vi "Measurement Logic.vi"() -> ()   [LabVIEW 2022 SP3, in "Calibrate Acoustic Output Level.lvlib"]
uses:
  Calibrate Acoustic Output Level.lvlib
  <vilib>/Plug-In SDKs/Measurements/Measure Call Context/Measure Call Context.lvclass
  Measurement Configuration.ctl
  Measurement Results.ctl
  <vilib>/addons/_NISVFA/_Generation/Signal Generation/SV Signal/sv_System Timing Model.ctl
  <vilib>/DAQmx/write.llb/DAQmx Write (Analog Wfm 1Chan NSamp).vi
  <vilib>/Analysis/1siggen.llb/Ramp Pattern by Samples.vi
  <vilib>/addons/_NISVFA/_Generation/Signal Generation/SV Sinusoid/SV Sinusoid.lvclass
  C:/Program Files/National Instruments/LabVIEW 2022/vi.lib/addons/_NISVFA/_Generation/Signal Generation/SV Signal/SV Signal.lvclass
  <vilib>/addons/_NISVFA/_Generation/Signal Generation/SV Sinusoid/Configure Sine.vi
  <vilib>/DAQmx/create/channels.llb/DAQmx Create Channel (AO-Voltage-Basic).vi
  <vilib>/DAQmx/configure/timing.llb/DAQmx Timing (Sample Clock).vi
  <vilib>/addons/_NISVFA/_Generation/Signal Generation/SV Signal/Write Sample Rate.vi
  <vilib>/addons/_NISVFA/_Generation/Signal Generation/SV Signal/Write System Timing Model.vi
  <vilib>/addons/_NISVFA/_Generation/Signal Generation/SV Signal/Write Ramp Parameters.vi
  <vilib>/DAQmx/miscellaneous.llb/DAQmx Fill In Error Info.vi
  <vilib>/DAQmx/create/channels.llb/DAQmx Create Channel (AI-Sound Pressure-Microphone).vi
  <vilib>/addons/_NISVFA/_Generation/Signal Generation/SV Signal/SV Signal.lvclass
  <vilib>/addons/Sound and Vibration/svt_Level/SoundVib_SoundLevel.lvlib
  <resource>/objmgr/daqmx.rc
  <vilib>/Analysis/NI_AALBase.lvlib
  <vilib>/gmath/NI_Gmath.lvlib
  <vilib>/addons/Sound and Vibration/svt_Level/SVL Leq Sound Level (1 Ch).vi
  <vilib>/DAQmx/read.llb/DAQmx Read (Analog Wfm 1Chan NSamp).vi
panel:
  out "crossed":bool=TRUE
  out "output voltage ratio":dbl=3.3942875477425276 format="%#_g Pa/Vpk"
  out "Waveform Graph":waveform(dbl)(graph)={"t0"=timestamp(3812465362.0113354 s since 1904-01-01), "dt"=1.9531249997269942e-05, "Y"=array[12800 elements], "attributes"=variant("NI_ChannelName"=variant(string "PXI1Slot2/ai0"), "NI_UnitDescription"=variant(string "Pascals"), "NI_dBReference"=variant(dbl 2e-05))}
  out "dBSPL":dbl=98.44719956931596
  out "measurement results":T1
  in  "measurement configuration":T2={"output channel"="Lorem ipsum dolor sit", "target value (dB)"=1.2, "number of steps"=32.0, "start amplitude (Vpk)"=32.0, "stop amplitude (Vpk)"=64.0, "frequency"=64.0, "ref mic channel"="PXI1Slot3\\ai0", "ref mic sensitivity (mV/Pa)"=-32.0} {"stop amplitude (Vpk)" format="%#_3f"; "start amplitude (Vpk)" format="%#.3f"}
  out "measure call context out":refnum<class "Measure Call Context.lvclass">
  in  "measure call context in":refnum<class "Measure Call Context.lvclass">
  out "error out":errorcluster
  in  "error in":errorcluster
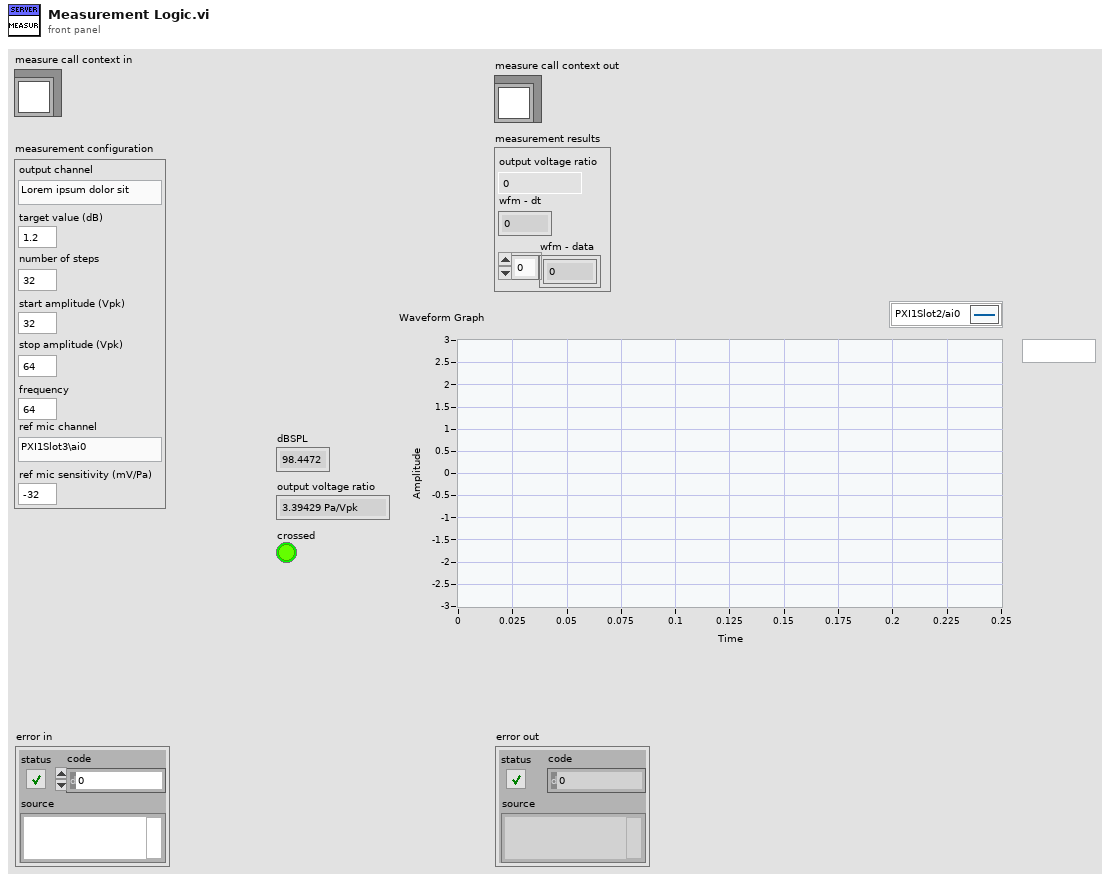
[diagram p1: front panel]
types:
  T1 = typedef "Calibrate Acoustic Output Level.lvlib/Measurement Results.ctl" = cluster{"output voltage ratio":dbl, "wfm - dt":dbl, "wfm - data":dbl[]}
  T2 = typedef "Calibrate Acoustic Output Level.lvlib/Measurement Configuration.ctl" = cluster{"output channel":string, "target value (dB)":dbl, "number of steps":dbl, "start amplitude (Vpk)":dbl, "stop amplitude (Vpk)":dbl, "frequency":dbl, "ref mic channel":string, "ref mic sensitivity (mV/Pa)":dbl}
  T3 = typedef "SV Signal.lvclass/sv_System Timing Model.ctl" = i64
  T4 = cluster{"profile":enum16{"Linear", "Half cosine"}, "durations [s]":cluster{"ramp-up":dbl, "transition":dbl, "ramp-down":dbl}}
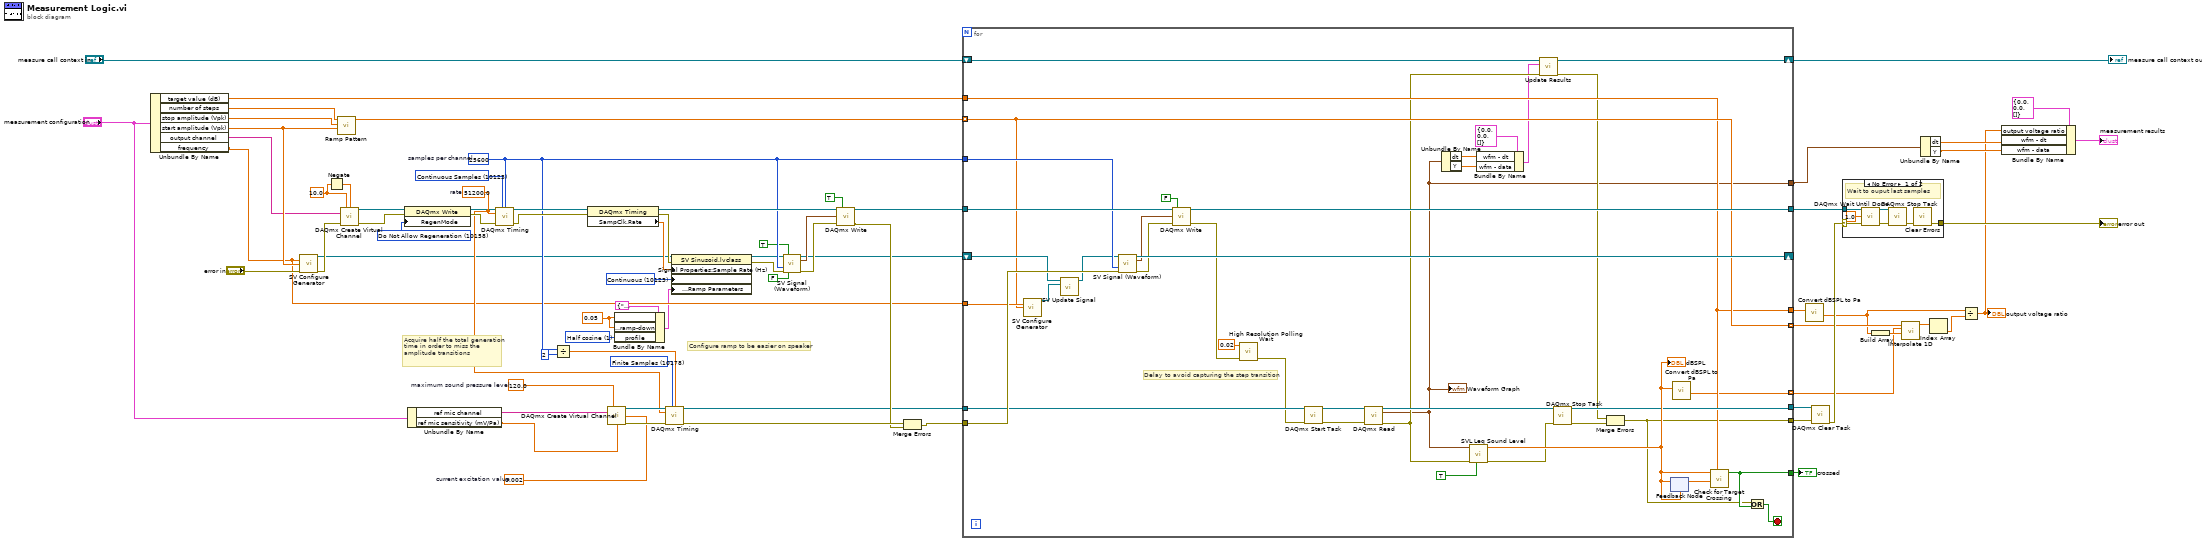
[diagram p0: block diagram]
diagram:
  w8 = 0.05 ("ramp duration")
  w6 = u16 1 items=["Linear", "Half cosine"] ("ramp profile")
  w5 = T3 10123 items=["Finite"=10178, "-"=-1, "Continuous"=10123, "-"=-2, "Settled"=110123, "Averaged"=210123, "Discrete Sweep"=310123, "Continuous Sweep"=410123] ("System Timing Model")
  w51 = 0.002  # current excitation value
  w54 = 120.0  # maximum sound pressure level
  w55 = 10178 items=["Finite Samples"=10178, "Continuous Samples"=10123] ("sample mode")
  w62 = 10158 items=["Allow Regeneration"=10097, "Do Not Allow Regeneration"=10158] ("RegenMode")
  w66 = 10.0 ("maximum value")
  w37 = 25600  # samples per channel
  w68 = 10123 items=["Finite Samples"=10178, "Continuous Samples"=10123, "Hardware Timed Single Point"=12522] ("sample mode")
  w42 = 51200.0  # rate
  # "Configure ramp to be easier on speaker"
  # "Acquire half the total generation time in order to miss the amplitude transitions"
  n1 = Unbundle By Name("measurement configuration") -> ("target value (dB)"=w25:dbl, "number of steps"=w24:dbl, "stop amplitude (Vpk)"=w23:dbl, "start amplitude (Vpk)"=w22:dbl, "output channel"=w21:string, "frequency"=w20:dbl)
  n2 = call-poly <vilib>:"SV Configure Generator.vi"("frequency (Hz)"=w20, "amplitude"=w22, "error in (no error)"="error in") -> ("signal configuration"=w11:refnum<class "SV Sinusoid.lvclass">, "error out"=w64:errorcluster)  [unwired: 11 in]
  n3 = Negate(x=w66) -> (-x=w65:dbl)
  n4 = call-poly <vilib>:"Ramp Pattern.vi"("start"=w22, "end"=w23, "samples"=w24) -> ("Ramp Pattern"=w41:dbl[])  [unwired: 7 in, 1 out]
  n5 = call-poly <vilib>:"DAQmx Create Virtual Channel.vi"("maximum value"=w66, "minimum value"=w65, "physical channels"=w21, "error in"=w64) -> ("task out"=w61:refnum<k21>, "error out"=w59:errorcluster)  [unwired: 10 in]
  n6 = property class="DAQmx Write"(reference=w61, error in=w59, "RegenMode"=w62) -> (reference out=w60:refnum<k21>, error out=w58:errorcluster)
  n7 = Unbundle By Name("measurement configuration") -> ("ref mic channel"=w19:string, "ref mic sensitivity (mV/Pa)"=w18:dbl)
  n8 = call-poly <vilib>:"DAQmx Timing.vi"("task/channels in"=w60, "sample mode"=w68, "samples per channel"=w37, "rate"=w42, "error in"=w58) -> ("task out"=w69:refnum<k21>, "error out"=w67:errorcluster)  [unwired: 9 in]
  n9 = Divide(x=w37, y=2) -> (x/y=w35:dbl)
  n10 = property class="DAQmx Timing"(reference=w69, error in=w67) -> (reference out=w48:refnum<k21>, error out=w56:errorcluster, "SampClk.Rate"=w57:dbl)
  n11 = call-poly <vilib>:"DAQmx Create Virtual Channel.vi"("maximum sound pressure level"=w54, "physical channels"=w19, "current excitation value"=w51, "microphone sensitivity"=w18) -> ("task out"=w53:refnum<k21>, "error out"=w52:errorcluster)  [unwired: 10 in]
  n12 = Bundle By Name(cluster=T4 {"profile"=enum."Linear", "durations [s]"={"ramp-up"=0.0, "transition"=0.0, "ramp-down"=0.0}} ("Ramp Parameters:All Elements"), "durations [s].ramp-up"=w8, "durations [s].ramp-down"=w8, "profile"=w6) -> (w7:T4)
  n13 = call-poly <vilib>:"DAQmx Timing.vi"("task/channels in"=w53, "sample mode"=w55, "samples per channel"=w35, "rate"=w42, "error in"=w52) -> ("task out"=w39:refnum<k21>, "error out"=w45:errorcluster)  [unwired: 9 in]
  n14 = property class="SV Sinusoid.lvclass"(reference=w11, error in=w56, "Signal Properties:Sample Rate (Hz)"=w57, "Signal Properties:System Timing Model"=w5, "Signal Properties:Ramps:Ramp Parameters"=w7) -> (reference out=w4:refnum<class "SV Sinusoid.lvclass">, error out=w3:errorcluster)
  n15 = call-dynamic "SV Signal (Waveform).vi"("signal configuration"=w4, "reset"=TRUE, "samples"=w37, "error in (no error)"=w3, "stop"=FALSE) -> ("signal configuration"=w10:refnum<class "SV Sinusoid.lvclass">, "output waveform"=w49:waveform(dbl), "error out"=w50:errorcluster)  [unwired: 5 in, 3 out]
  n16 = call-poly <vilib>:"DAQmx Write.vi"("task/channels in"=w48, "auto start"=TRUE, "data"=w49, "error in"=w50) -> ("task out"=w47:refnum<k21>, "error out"=w40:errorcluster)  [unwired: 9 in, 1 out]
  n17 = Merge Errors(w45, w40) -> (w38:errorcluster)
  n18 = for {
    shift-right: [w114] -> _
    shift-left: w10 -> [w105]
    tunnel: w37 -> [w108]
    tunnel: w47 -> [w113]
    tunnel: [w112] -> w63
    tunnel: w38 -> [w107]
    tunnel: w39 -> [w98]
    tunnel: [w94] -> w44
    tunnel: w20 -> [w103]
    tunnel: w41 -> [w89] mode=indexing
    tunnel: w25 -> [w88]
    tunnel: [w90] -> w28
    tunnel: [w89] -> w29 mode=indexing
    tunnel: [w87] -> w33 mode=indexing
    tunnel: [w88] -> w32
    shift-right: [w82] -> w71
    shift-left: "measure call context in" -> [w81]
    tunnel: [w76] -> w17
    tunnel: [w75] -> w12
    stop <- w101 stop-if-true
    # "Delay to avoid capturing the step transition"
    n19 = call-poly <vilib>:"SV Configure Generator.vi"("frequency (Hz)"=w103, "amplitude"=w89) -> ("signal configuration"=w106:refnum<class "SV Sinusoid.lvclass">)  [unwired: 12 in, 1 out]
    n20 = call-dynamic "SV Update Signal.vi"("current configuration"=w105, "new configuration"=w106) -> ("updated configuration"=w104:refnum<class "SV Sinusoid.lvclass">)  [unwired: 12 in, 1 out]
    n21 = call-dynamic "SV Signal (Waveform).vi"("signal configuration"=w104, "samples"=w108, "error in (no error)"=w107) -> ("signal configuration"=w114:refnum<class "SV Sinusoid.lvclass">, "output waveform"=w109:waveform(dbl), "error out"=w111:errorcluster)  [unwired: 7 in, 3 out]
    n22 = call-poly <vilib>:"DAQmx Write.vi"("task/channels in"=w113, "auto start"=FALSE, "data"=w109, "error in"=w111) -> ("task out"=w112:refnum<k21>, "error out"=w93:errorcluster)  [unwired: 9 in, 1 out]
    n23 = call <vilib>:"High Resolution Polling Wait.vi"("error in (no error)"=w93, "seconds to wait"=0.02) -> ("error out"=w92:errorcluster)  [unwired: 9 in]
    n24 = call <vilib>:"DAQmx Start Task.vi"("task/channels in"=w98, "error in"=w92) -> ("task out"=w97:refnum<k21>, "error out"=w96:errorcluster)  [unwired: 12 in]
    n25 = call-poly <vilib>:"DAQmx Read.vi"("task/channels in"=w97, "error in"=w96) -> ("task out"=w95:refnum<k21>, "data"=w76:waveform(dbl), "error out"=w85:errorcluster)  [unwired: 11 in]
    "Waveform Graph" <- w76
    n26 = Unbundle By Name(w76) -> ("dt"=w78:dbl, "Y"=w77:dbl[])
    n27 = call-poly <vilib>:"SVL Leq Sound Level.vi"("restart averaging (F)"=TRUE, "error in (no error)"=w85, "scaled signal [EU]"=w76) -> ("error out"=w86:errorcluster, "Leq sound level [dB EU]"=w99:dbl)  [unwired: 6 in, 1 out]
    "dBSPL" <- w99
    n28 = Bundle By Name(cluster=T1 {"output voltage ratio"=0.0, "wfm - dt"=0.0, "wfm - data"=[]} ("Measurement Results"), "wfm - dt"=w78, "wfm - data"=w77) -> (w79:T1)
    n29 = call <vilib>:"Update Results.vi"("error in"=w85, "measurement results"=w79, "measure call context in"=w81) -> ("error out"=w83:errorcluster, "measure call context out"=w82:refnum<class "Measure Call Context.lvclass">)  [unwired: 7 in]
    n30 = call <vilib>:"DAQmx Stop Task.vi"("task/channels in"=w95, "error in"=w86) -> ("task out"=w94:refnum<k21>, "error out"=w84:errorcluster)  [unwired: 12 in]
    n31 = Merge Errors(w83, w84) -> (w75:errorcluster)
    n32 = feedback-in #1(w99) -> ()
    n33 = feedback #1(w99) -> (w100:dbl)
    n34 = call "Convert dBSPL to Pa.vi"("dB SPL"=w99) -> ("Pa pk"=w87:dbl)  [unwired: 9 in, 1 out]
    n35 = call "Check for Target Crossing.vi"("target value"=w88, "previous value"=w100, "current value"=w99) -> ("crossed"=w90:bool)  [unwired: 8 in]
    n36 = Or(x=w75, y=w90) -> (x .or. y?=w101:bool)
  }
  "measure call context out" <- w71
  "crossed" <- w28
  n37 = call "Convert dBSPL to Pa.vi"("dB SPL"=w32) -> ("Pa pk"=w27:dbl)  [unwired: 9 in, 1 out]
  n38 = call <vilib>:"DAQmx Clear Task.vi"("task in"=w44, "error in"=w12) -> ("error out"=w43:errorcluster)  [unwired: 13 in]
  n39 = case shown="No Error" w43 {
    selector: w43 -> [w118 w122]
    tunnel: w63 -> [w121 _]
    tunnel: [w115 w122] -> w74
    frame No Error {
      # "Wait to ouput last samples"
      n40 = call <vilib>:"DAQmx Wait Until Done.vi"("task/channels in"=w121, "timeout (sec)"=1.0, "error in"=w118) -> ("task out"=w120:refnum<k21>, "error out"=w119:errorcluster)  [unwired: 11 in]
      n41 = call <vilib>:"DAQmx Stop Task.vi"("task/channels in"=w120, "error in"=w119) -> ("error out"=w116:errorcluster)  [unwired: 12 in, 1 out]
      n42 = call <vilib>:"Clear Errors.vi"("error in (no error)"=w116) -> ("error out"=w115:errorcluster)  [unwired: 5 in, 1 out]
    }
    frame Error {
      # "Error"
    }
  }
  "error out" <- w74
  n43 = Build Array(w27) -> (w34:dbl[])
  n44 = call <vilib>:"Interpolate 1D.vi"("xi"=w34, "X"=w33, "Y"=w29) -> ("yi"=w31:dbl[])  [unwired: 6 in, 2 out]
  n45 = Unbundle By Name(w17) -> ("dt"=w15:dbl, "Y"=w14:dbl[])
  n46 = Index Array(array=w31) -> (element=w30:dbl)  [unwired: 1 in]
  n47 = Divide(x=w27, y=w30) -> (x/y=w13:dbl)
  "output voltage ratio" <- w13
  n48 = Bundle By Name(cluster=T1 {"output voltage ratio"=0.0, "wfm - dt"=0.0, "wfm - data"=[]} ("Measurement Results"), "output voltage ratio"=w13, "wfm - dt"=w15, "wfm - data"=w14) -> (→"measurement results":T1)
